vi "Create Fast Draw Object.vi"(6 "Actual Transform In":T1, 8 "error in (no error)":errorcluster, 9 "Multiplot Representation In":T3, 10 "3D Comet.lvclass in":refnum<class "3D Comet.lvclass">, 11 "Plot Object In":refnum<vi>) -> (0 "error out":errorcluster, 1 "Multiplot Representation Out":T3, 2 "3D Comet.lvclass out":refnum<class "3D Comet.lvclass">, 3 "Plot Object Out":refnum<vi>, 4 "Actual Transform Out":T1)   [LabVIEW 2020, in "3D Comet.lvclass"]
uses:
  <vilib>/Math Plots/3D Math Plots/3D Comet/3D Comet/3D Comet.lvclass
  <vilib>/Math Plots/3D Math Plots/3D Plot/3D Plot/Typedef/Multiplot Representation.ctl
  <vilib>/Math Plots/3D Math Plots/3D Plot/3D Plot/Typedef/Plot Representation.ctl
  <vilib>/Math Plots/3D Math Plots/3D Plot/3D Plot/Typedef/Range Clusters.ctl
  <vilib>/Math Plots/3D Math Plots/3D Plot/3D Plot/Typedef/Mesh Data.ctl
  <vilib>/Math Plots/3D Math Plots/3D Plot/3D Plot/Typedef/Actual Transform.ctl
  <vilib>/Math Plots/3D Math Plots/3D Comet/3D Comet/3D Comet.lvclass/3D Comet.ctl
  <vilib>/Math Plots/3D Math Plots/3D Plot/3D Plot/3D Plot.lvclass
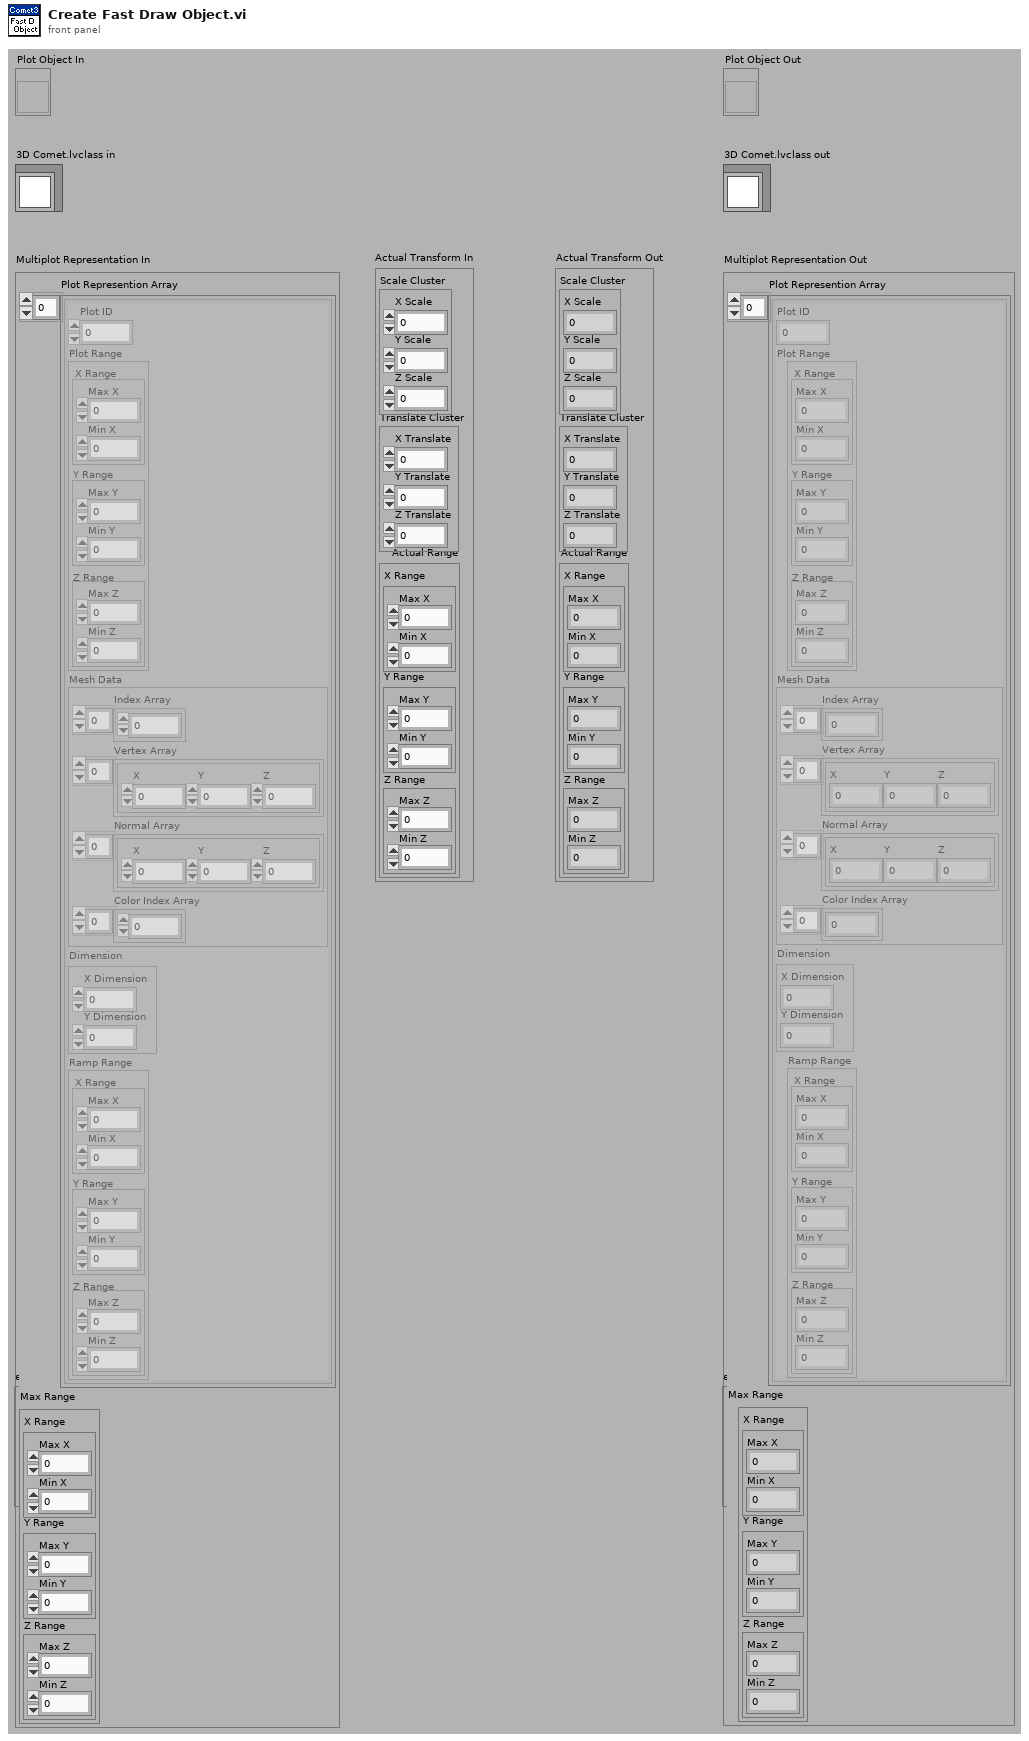
[diagram p1: front panel]
types:
  T1 = typedef "3D Plot.lvclass/Actual Transform.ctl" = cluster{"Scale Cluster":cluster{"X Scale":sgl, "Y Scale":sgl, "Z Scale":sgl}, "Translate Cluster":cluster{"X Translate":sgl, "Y Translate":sgl, "Z Translate":sgl}, "Actual Range":T2}
  T2 = typedef "3D Plot.lvclass/Range Clusters.ctl" = cluster{"X Range":cluster{"Max X":sgl, "Min X":sgl}, "Y Range":cluster{"Max Y":sgl, "Min Y":sgl}, "Z Range":cluster{"Max Z":sgl, "Min Z":sgl}}
  T3 = typedef "3D Plot.lvclass/Multiplot Representation.ctl" = cluster{"Plot Represention Array":T4[], "Max Range":T2}
  T4 = typedef "3D Plot.lvclass/Plot Representation.ctl" = cluster{"Plot ID":i32, "Plot Range":T2, "Mesh Data":T5, "Dimension":cluster{"X Dimension":i32, "Y Dimension":i32}, "Ramp Range":T2}
  T5 = typedef "3D Plot.lvclass/Mesh Data.ctl" = cluster{"Index Array":u32[], "Vertex Array":cluster{"X":sgl, "Y":sgl, "Z":sgl}[], "Normal Array":cluster{"X":sgl, "Y":sgl, "Z":sgl}[], "Color Index Array":i32[]}
  T6 = typedef "3D Comet.lvclass/3D Comet Property Array.ctl" = T7[]
  T7 = typedef "3D Comet.lvclass/3D Comet Property.ctl" = cluster{"General Property":cluster{"Plot Name":string, "Coordinate System":enum16{"Cartesian", "Cylindrical", "Spherical"}, "Opacity":sgl}, "Projection Property":cluster{"Draw XY":bool, "Draw YZ":bool, "Draw XZ":bool}, "Plot Property":cluster{"Sprite Type":T8, "Point Size":sgl, "Point Color":u32, "Line Style":T9, "Line Width":sgl, "Line Color":u32, "Antialiasing":bool}, "Comet Property":cluster{"Body length":sgl}}
  T8 = typedef "3D Plot.lvclass/Sprite Type.ctl" = enum16{"None", "Empty Square", "Solid Square", "Empty Diamond", "Solid Diamond", "Empty Circle", "Solid Circle", "Asterisk", "Bold X", "Wireframe Sphere", "Solid Sphere", "Wireframe Cube", "Solid Cube"}
  T9 = typedef "3D Plot.lvclass/Line Type.ctl" = enum16{"None", "Solid", "Dash", "Dot", "Dash Dot"}
  T10 = enum16{"Points", "Lines", "Line Strip", "Line Loop", "Triangles", "Triangle Strip", "Triangle Fan", "Quads", "Quad Strip", "Polygon"}
  T11 = cluster{"Draw XY":bool, "Draw YZ":bool, "Draw XZ":bool}
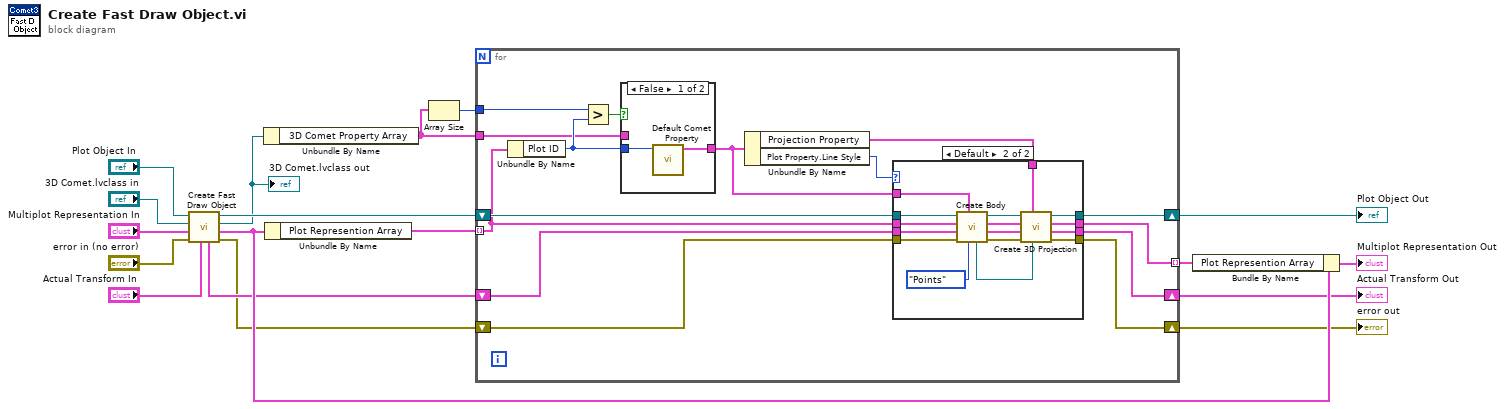
[diagram p0: block diagram]
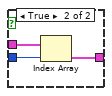
[diagram p2: hidden frame]
diagram:
  n1 = call-parent "Create Fast Draw Object.vi"("Actual Transform In"="Actual Transform In", "error in (no error)"="error in (no error)", "Multiplot Representation In"="Multiplot Representation In", "3D Plot.lvclass in"="3D Comet.lvclass in", "Plot Object In"="Plot Object In") -> ("error out"=w6:errorcluster, "Multiplot Representation Out"=w10:T3, "3D Plot.lvclass out"=w7:refnum<class "3D Comet.lvclass">, "Plot Object Out"=w11:refnum<vi>, "Actual Transform Out"=w9:T1)  [unwired: 2 out]
  "3D Comet.lvclass out" <- w7
  n2 = Unbundle By Name(w7) -> ("3D Comet Property Array"=w2:T6)
  n3 = Unbundle By Name(w10) -> ("Plot Represention Array"=w13:T4[])
  n4 = Array Size(array=w2) -> (size(s)=w1:i32)
  n5 = for {
    tunnel: w2 -> [w21]
    tunnel: w13 -> [w32] mode=indexing
    tunnel: [w25] -> w12 mode=indexing
    shift-right: [w28] -> w5
    shift-left: w9 -> [w31]
    shift-right: [w27] -> w3
    shift-left: w6 -> [w30]
    shift-right: [w29] -> w4
    shift-left: w11 -> [w33]
    tunnel: w1 -> [w19]
    n6 = Unbundle By Name(w32) -> ("Plot ID"=w22:i32)
    n7 = Greater?(x=w19, y=w22) -> (0:w23:bool)
    n8 = case shown="False" w23 {
      tunnel: w21 -> [_ w38]
      tunnel: [w34 w37] -> w20
      tunnel: w22 -> [w35 w36]
      frame False {
        n9 = call <vilib>:"Default Comet Property.vi"("Plot ID"=w35) -> ("Default Property"=w34:T7)  [unwired: 10 out]
      }
      frame True {
        n10 = Index Array(array=w38, index=w36) -> (element=w37:T7)
      }
    }
    n11 = Unbundle By Name(w20) -> ("Projection Property"=w26:T11, "Plot Property.Line Style"=w24:T9)
    n12 = case shown="Default" w24 {
      tunnel: w33 -> [w42 w57]
      tunnel: w32 -> [w39 w56]
      tunnel: w31 -> [w41 w55]
      tunnel: w30 -> [w40 w54]
      tunnel: [w42 w52] -> w29
      tunnel: [w41 w50] -> w28
      tunnel: [w40 w48] -> w27
      tunnel: w26 -> [_ w46]
      tunnel: w20 -> [_ w44]
      tunnel: [w39 w43] -> w25
      frame "None" {
      }
      frame Default {
        n13 = call <vilib>:"Create Body.vi"("Draw Mode"=T10."Points", "3D Comet Property"=w44, "error in (no error)"=w54, "Actual Transform In"=w55, "Plot Representation In"=w56, "Plot Object In"=w57) -> ("error out"=w49:errorcluster, "Actual Transform Out"=w51:T1, "Plot Representation Out"=w43:T4, "Plot Object Out"=w53:refnum<vi>, "Track Object Out"=w47:refnum<vi>)  [unwired: 1 in]
        n14 = call <vilib>:"Create 3D Projection.vi"("Sub Object In"=w47, "Projection Property"=w46, "error in (no error)"=w49, "Actual Transform In"=w51, "Plot Object In"=w53) -> ("error out"=w48:errorcluster, "Actual Transform Out"=w50:T1, "Plot Object Out"=w52:refnum<vi>)  [unwired: 1 in, 3 out]
      }
    }
  }
  "error out" <- w3
  "Plot Object Out" <- w4
  "Actual Transform Out" <- w5
  n15 = Bundle By Name(cluster=w10, "Plot Represention Array"=w12) -> (→"Multiplot Representation Out":T3)
